vi "外观 2.vi"(0 "Data In":T6 caption="数据输入" format="%04x", 2 "Display State In":T4 caption="显示状态输入", 3 "Container State":T5 caption="容器状态") -> (6 "Data Out":T6 caption="数据输出" format="%04x", 7 "Display State Out":T4 caption="显示状态输出", 8 "Action":T3 caption="动作")   [LabVIEW 2016, in "氨氮调试控件.xctl"]
uses:
  <vilib>/_xctls/Container State.ctl
  <vilib>/_xctls/Action.ctl
  <vilib>/_xctls/XControlSupport.lvlib
panel:
  out "选项卡控件":enum32{"选项卡 1", "选项卡 2"}(tab)
  in  "V9-2":bool
  in  "V9-1":bool
  in  "阀口选择":T1(radio)
  in  "外设":enum32{"未选择", "蠕动泵", "电磁阀1", "电磁阀2", "氨氮控温"}(radio)
  in  "控温":enum32{"未选择", "消解", "恒温", "降温"}(radio)
  in  "灯":enum32{"未选择", "365", "520", "660", "氙灯/紫灯"}(radio)
  in  "ADC值":T2(radio)
  in  "项目输入":enum32{"总磷", "总氮", "氨氮"}(ring)
  in  "功能选择":enum32{"等待", "复位", "注入", "注出"}(radio)=enum."注入"
  in  "数值":i16=4000
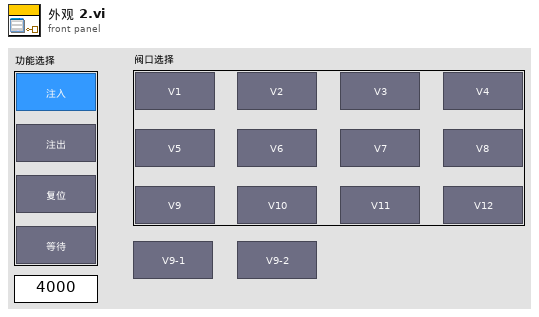
[diagram p1: front panel]
types:
  T1 = enum32{"未选择", "V1", "V2", "V3", "V4", "V5", "V6", "V7", "V8", "V9", "V10", "V11", "V12"}
  T2 = enum32{"未选择", "ADC365", "ADC520", "ADC660", "光谱仪"}
  T3 = typedef "XControlSupport.lvlib/Action.ctl" = cluster{"Data Changed?":bool, "State Changed?":bool, "Action Name":string}
  T4 = typedef "氨氮调试控件.xctl/状态 2.ctl" = cluster{"Numeric":dbl}
  T5 = typedef "XControlSupport.lvlib/Container State.ctl" = cluster{"Indicator?":bool, "Run Mode?":bool, " Refnum":refnum<vi>}
  T6 = typedef "氨氮调试控件.xctl/数据 2.ctl" = u16[]
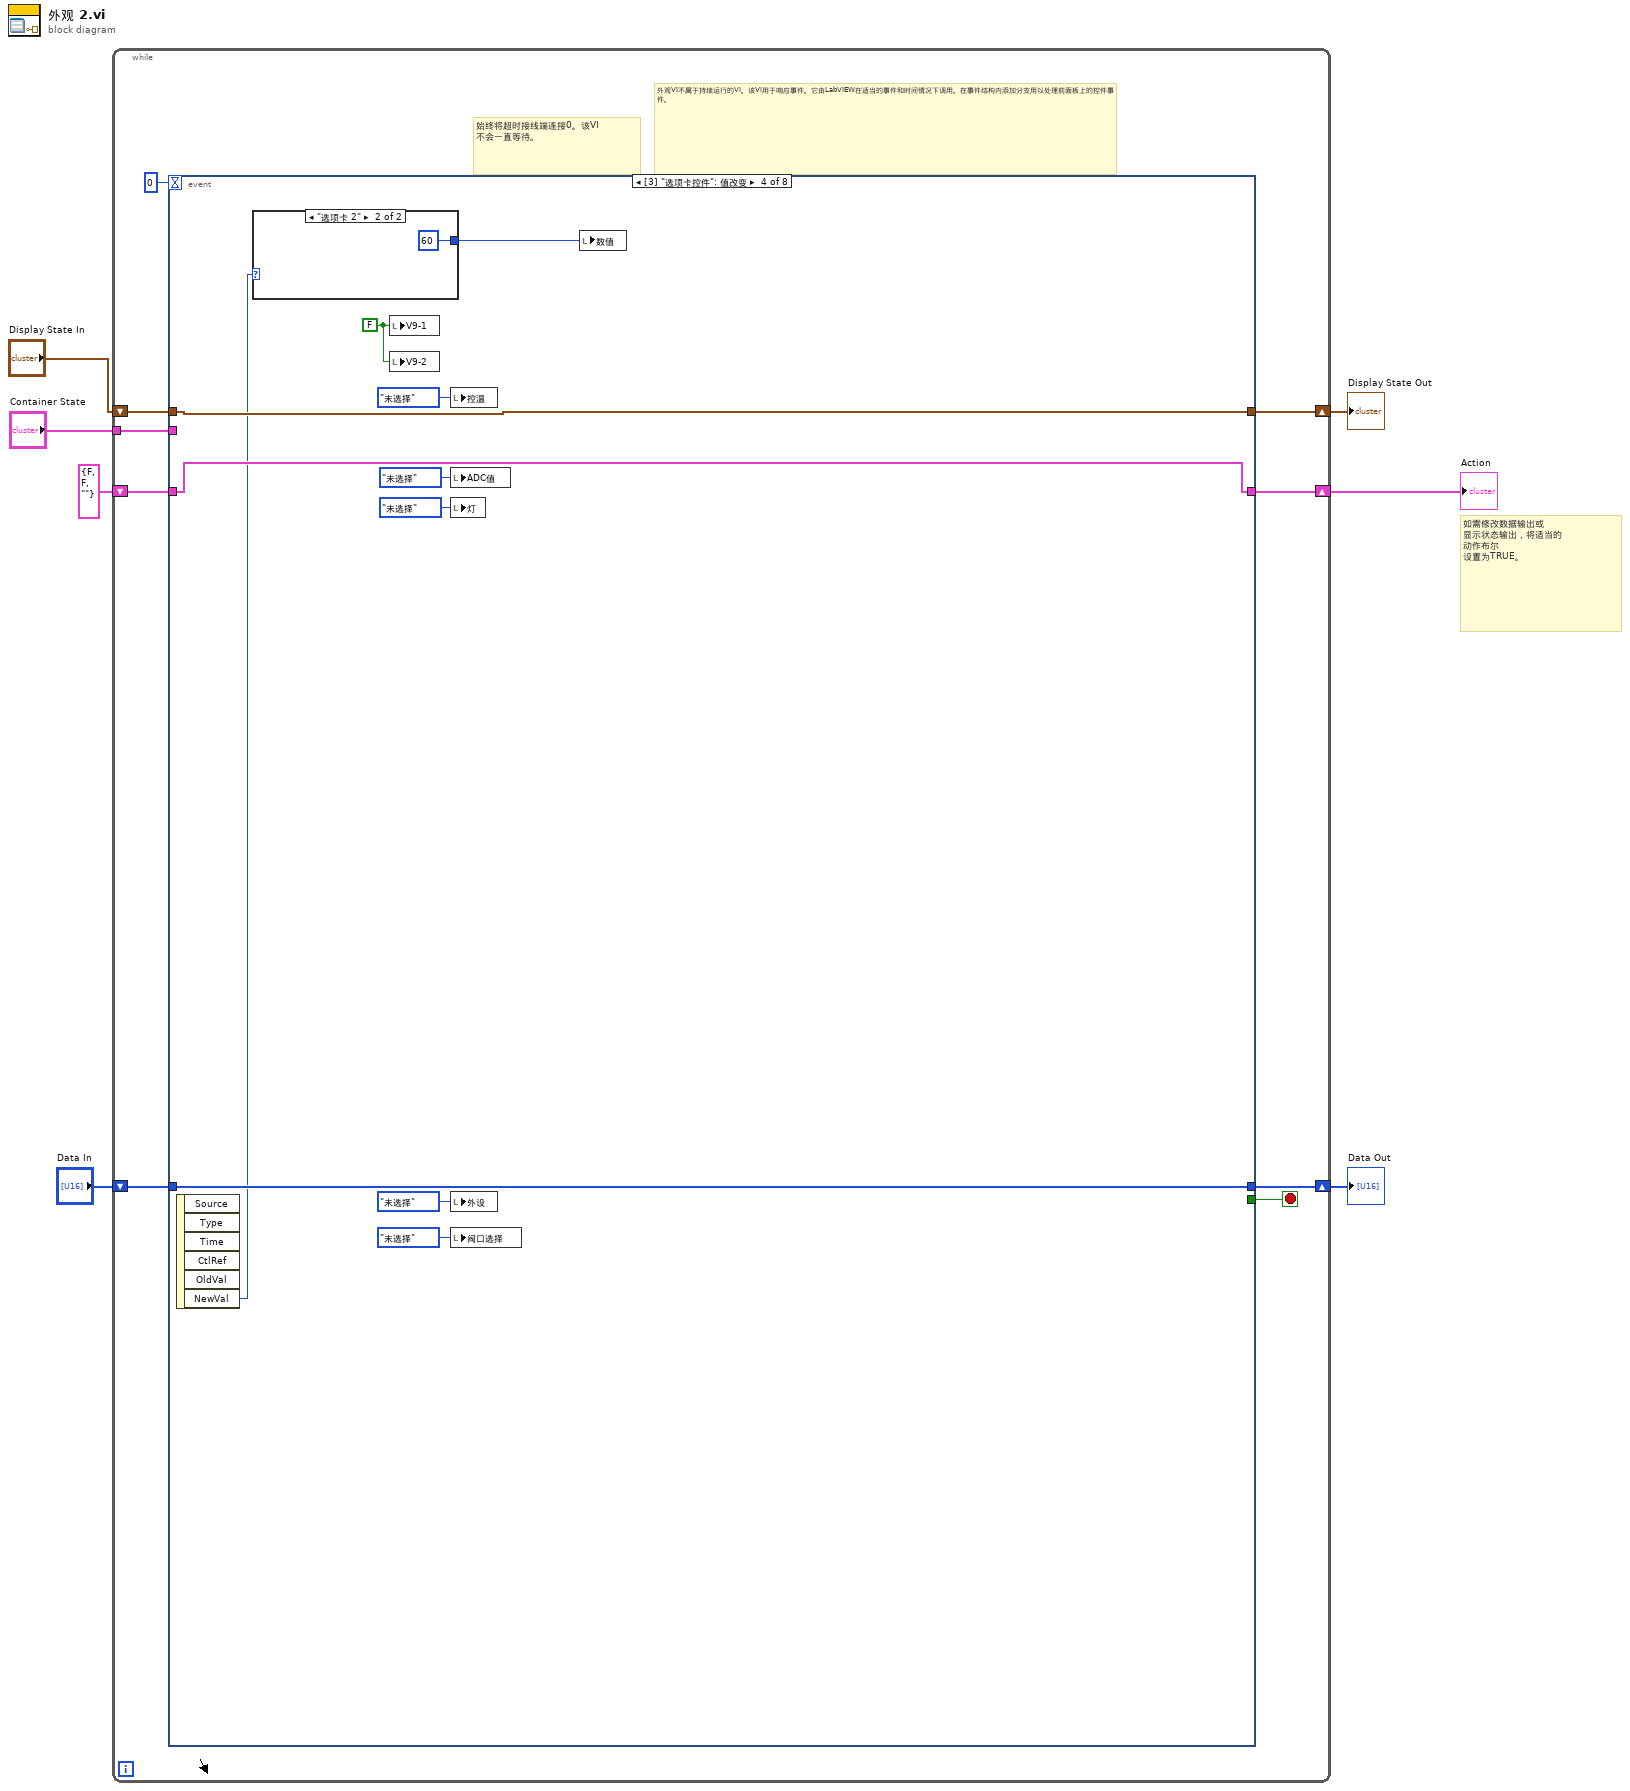
[diagram p0: block diagram]
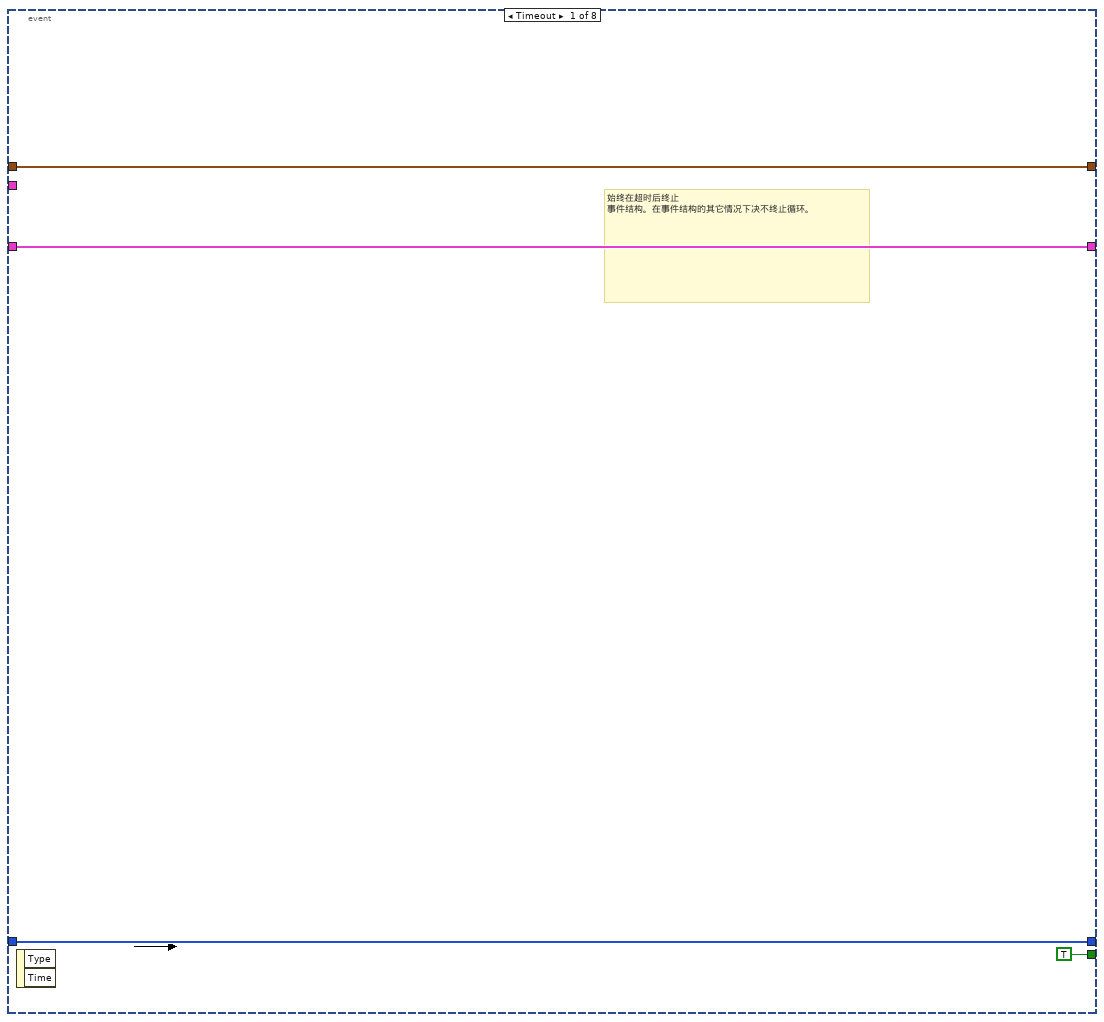
[diagram p2: hidden frame]
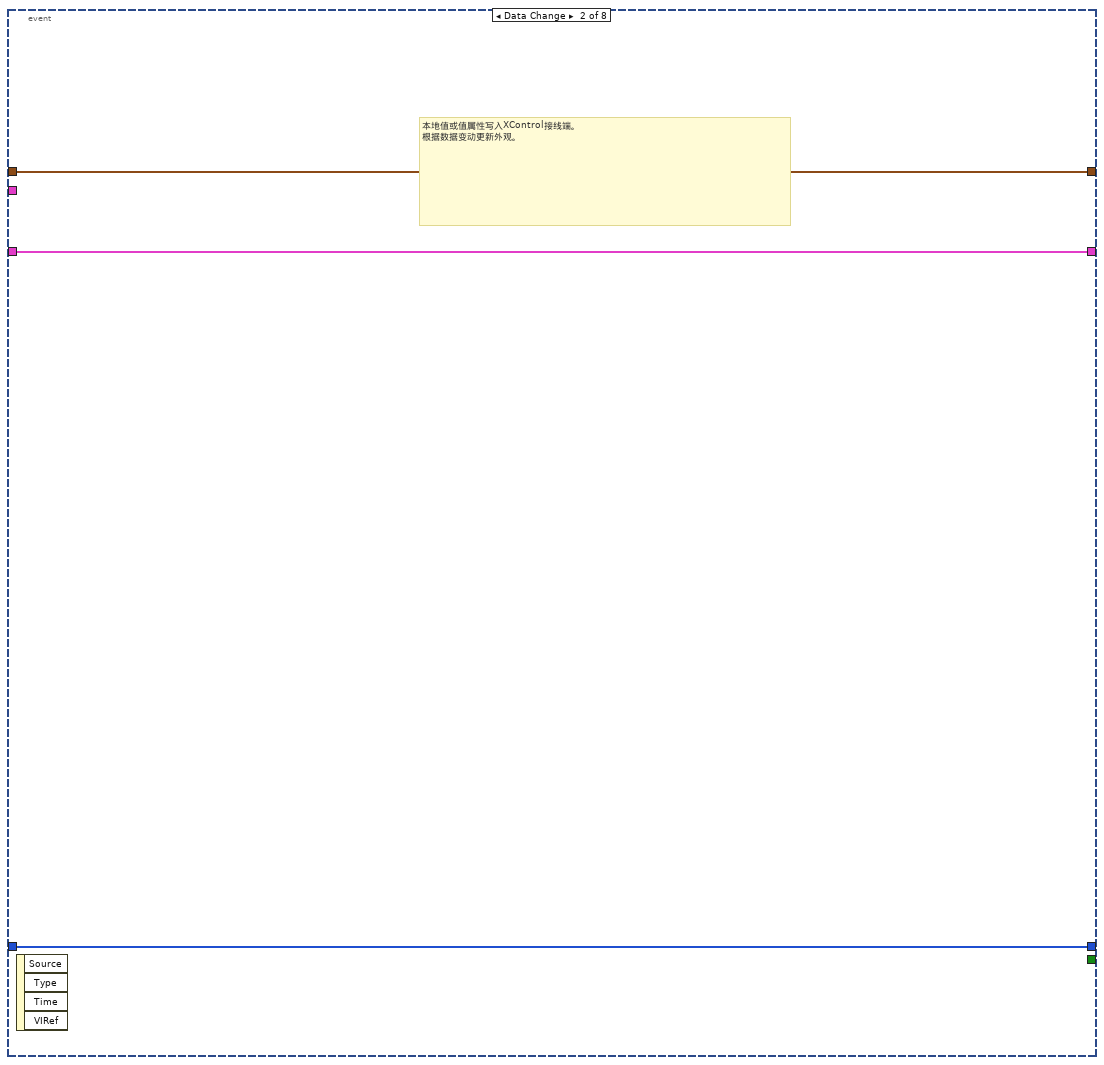
[diagram p3: hidden frame]
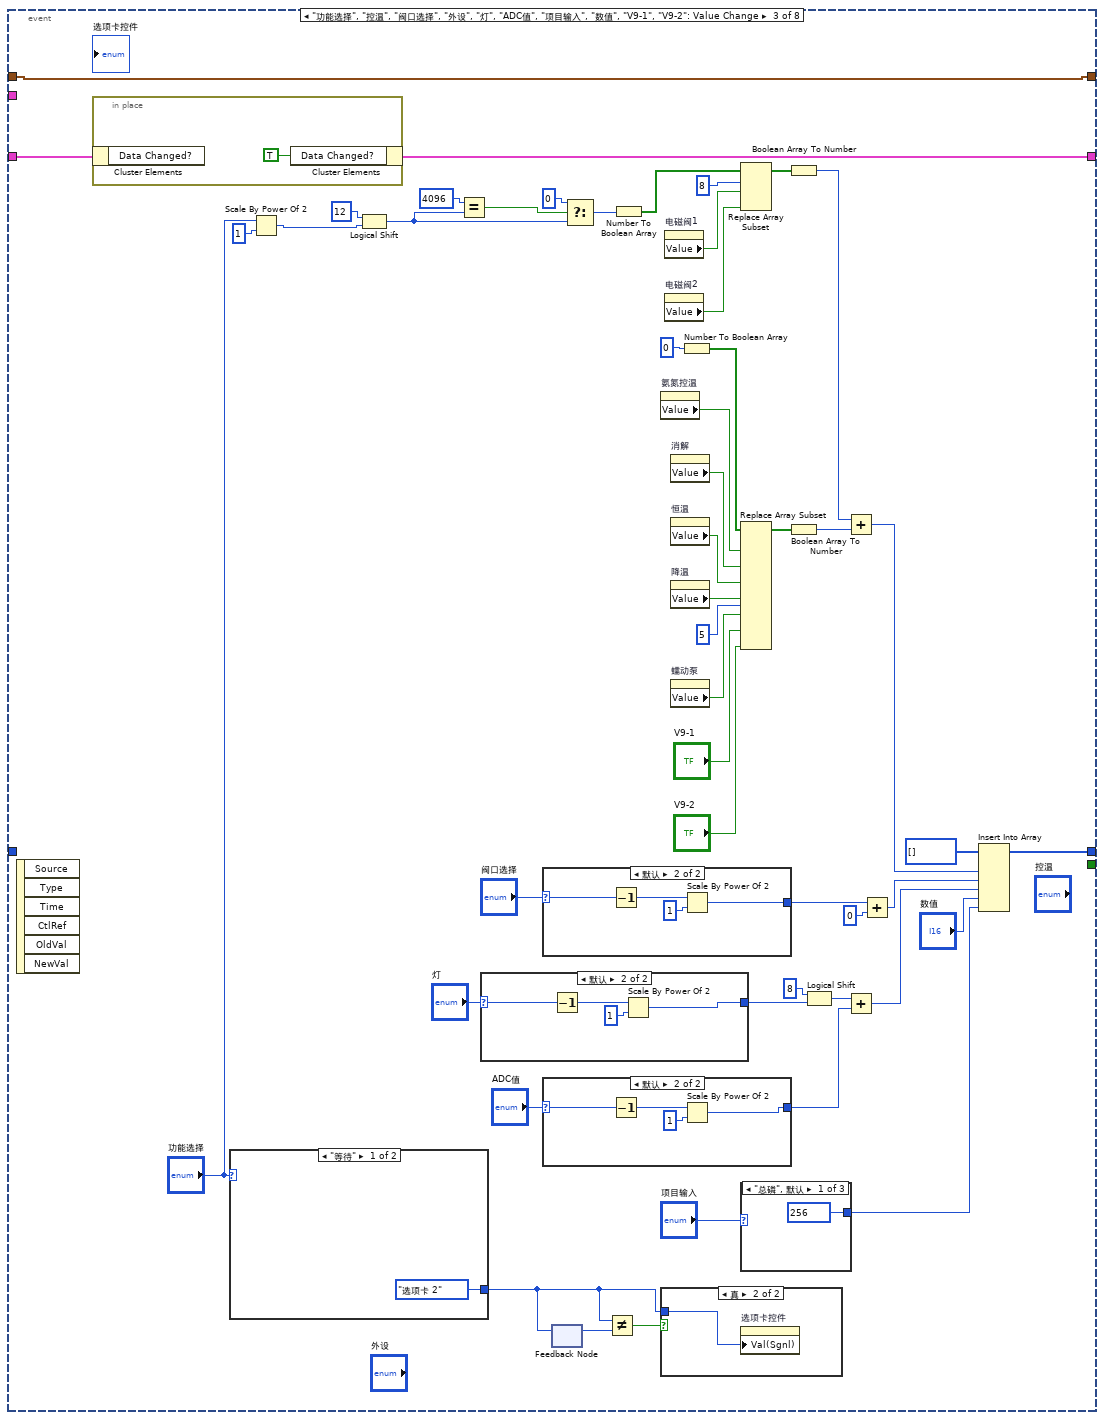
[diagram p4: hidden frame]
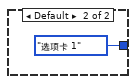
[diagram p6: hidden frame]
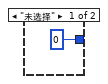
[diagram p7: hidden frame]
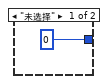
[diagram p8: hidden frame]
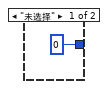
[diagram p9: hidden frame]
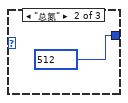
[diagram p10: hidden frame]
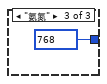
[diagram p11: hidden frame]
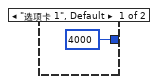
[diagram p12: hidden frame]
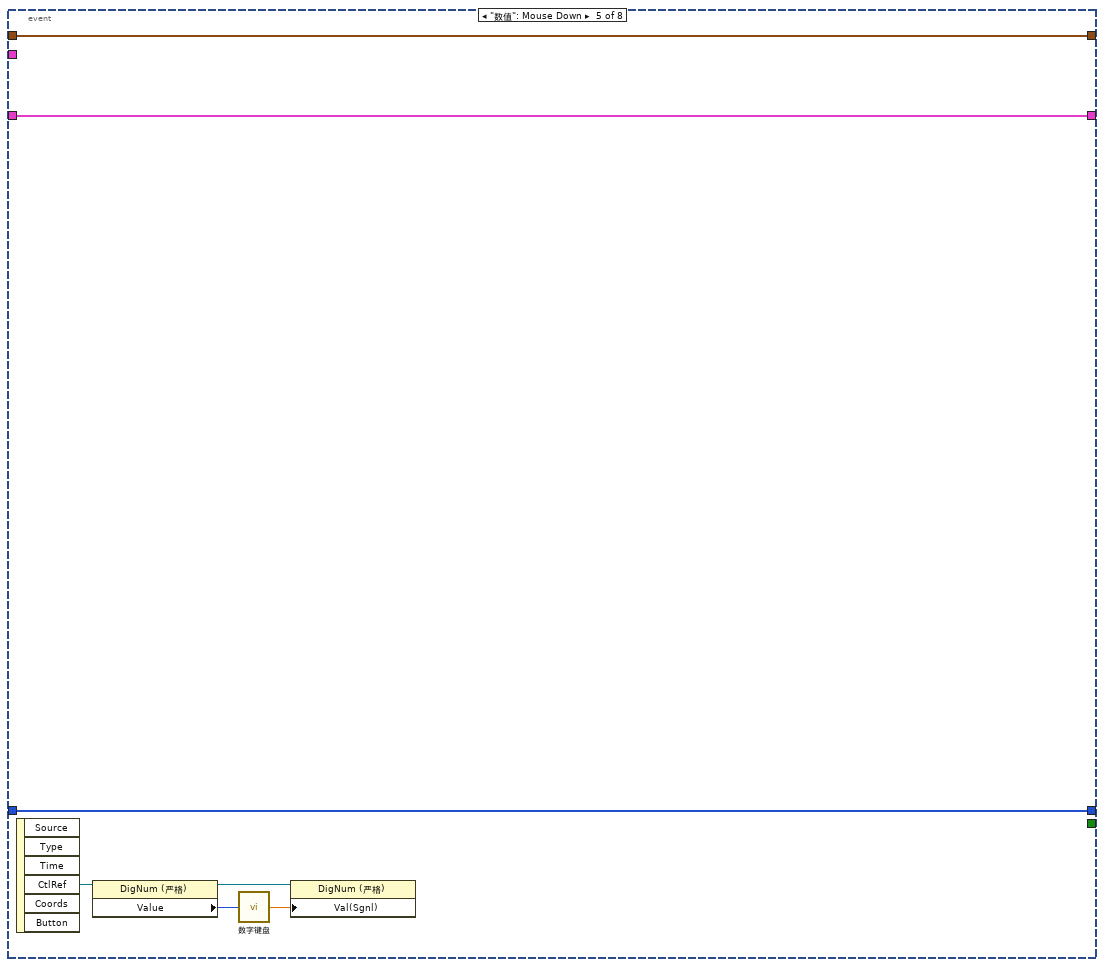
[diagram p13: hidden frame]
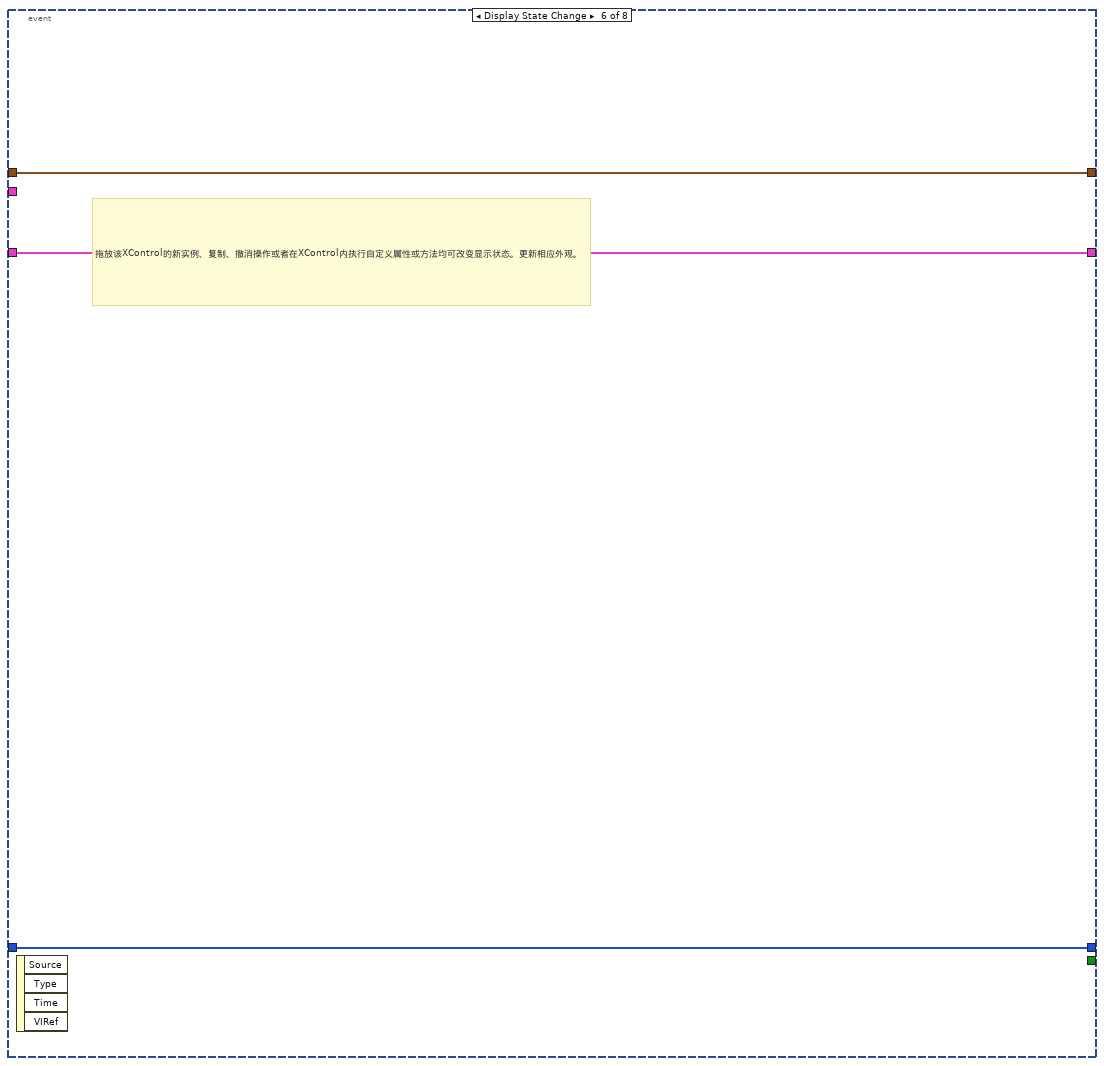
[diagram p14: hidden frame]
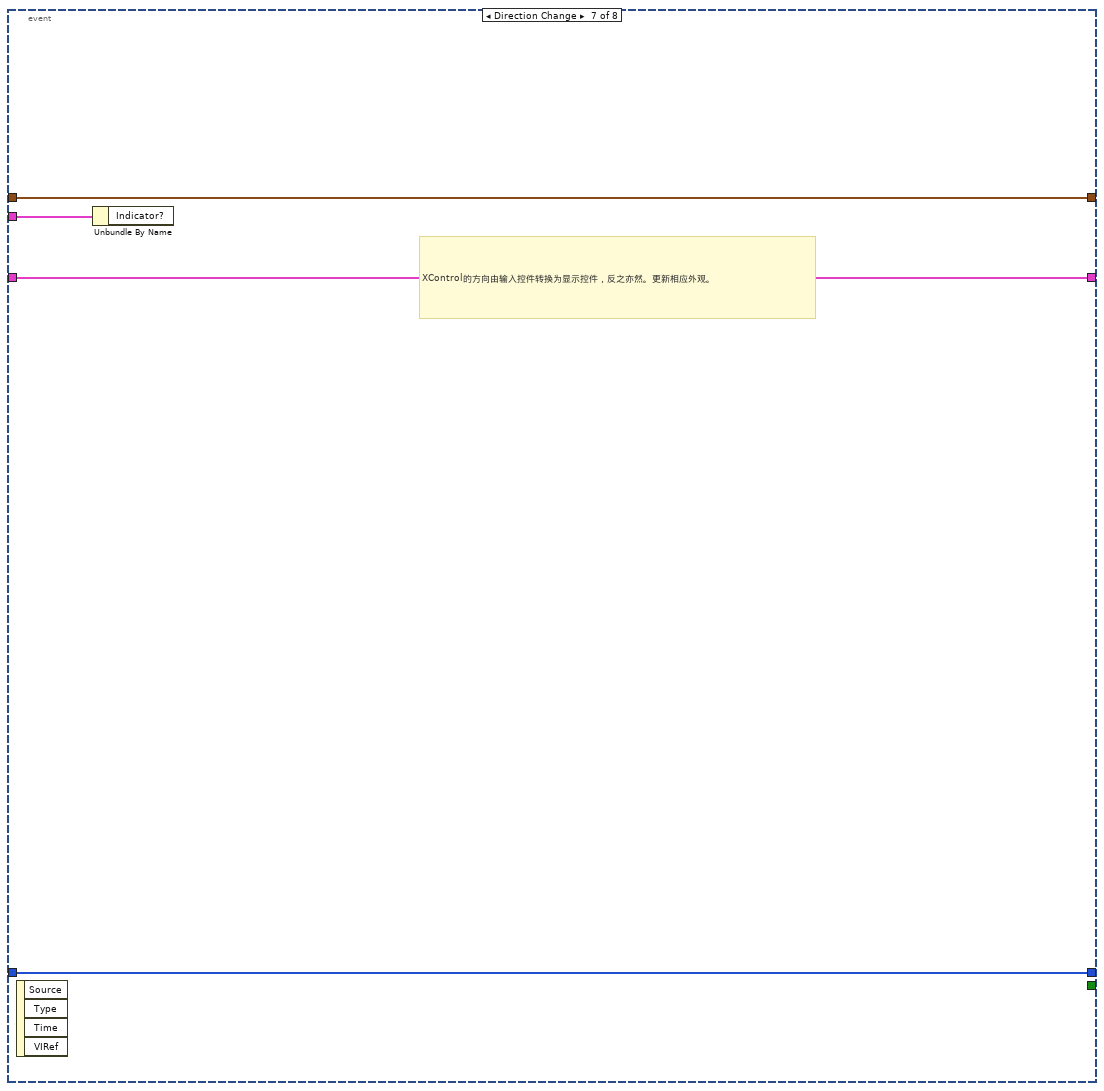
[diagram p15: hidden frame]
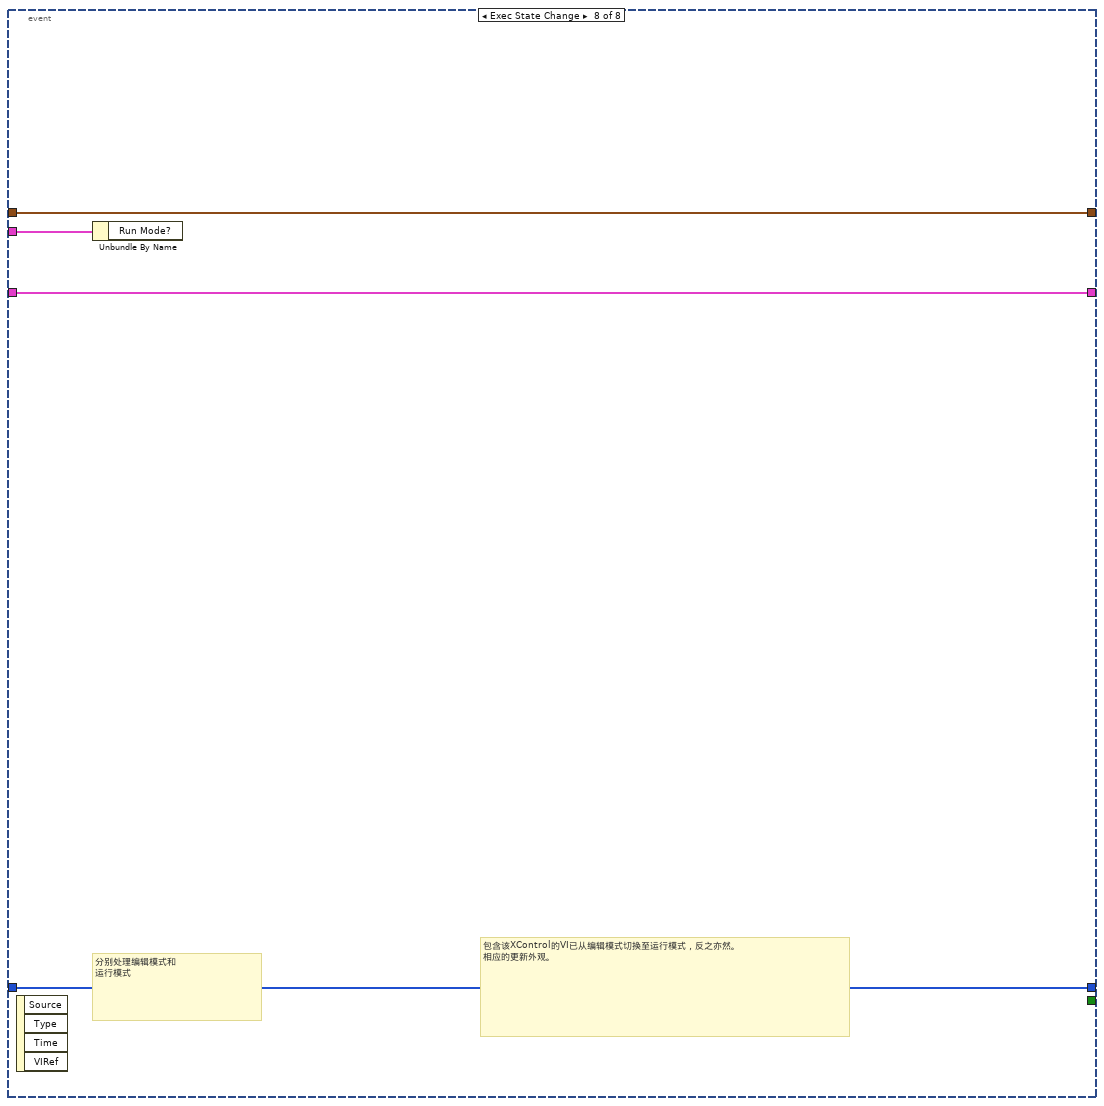
[diagram p16: hidden frame]
diagram:
  # "如需修改数据输出或\n显示状态输出，将适当的\n动作布尔\n设置为TRUE。"
  n1 = while {
    shift-right: [w15] -> w4
    shift-left: "Display State In" -> [w16]
    tunnel: "Container State" -> [w12]
    shift-right: [w10] -> w7
    shift-left: "Data In" -> [w11]
    shift-right: [w8] -> w2
    shift-left: T3 {"Data Changed?"=FALSE, "State Changed?"=FALSE, "Action Name"=""} ("Action") -> [w9]
    stop <- w14 stop-if-true
    # "外观VI不属于持续运行的VI。该VI用于响应事件。它由LabVIEW在适当的事件和时间情况下调用。在事件结构内添加分支用以处理前面板上的控件事件。"
    # "始终将超时接线端连接0。该VI\n不会一直等待。"
    n2 = event shown="[3] \"选项卡控件\": 值改变" {
      selector: _ -> [_ _ _ _ _ _ _ _]
      dyn-events: _ -> [_ _ _ _ _ _ _ _]
      timeout: 0 -> [_ _ _ _ _ _ _ _]
      tunnel: w16 -> [w18 w22 w73 w106 w115 w118 w121 w125]
      tunnel: [w18 w22 w73 w106 w115 w118 w121 w125] -> w15
      tunnel: [TRUE _ _ _ _ _ _ _] -> w14
      tunnel: w12 -> [_ _ _ _ _ _ w122 w126]
      tunnel: w11 -> [w17 w23 _ w105 w114 w117 w120 w124]
      tunnel: [w17 w23 w48 w105 w114 w117 w120 w124] -> w10
      tunnel: [w19 w21 w71 w104 w113 w116 w119 w123] -> w8
      tunnel: w9 -> [w19 w21 w72 w104 w113 w116 w119 w123]
      event Timeout {
        # "始终在超时后终止\n事件结构。在事件结构的其它情况下决不终止循环。"
        n3 = event-data() -> ()  [unwired: 1 in, 2 out]
      }
      event Data Change {
        # "本地值或值属性写入XControl接线端。\n根据数据变动更新外观。"
        n4 = event-data() -> ()  [unwired: 1 in, 4 out]
      }
      event "功能选择", "控温", "阀口选择", "外设", "灯", "ADC值", "项目输入", "数值", "V9-1", "V9-2": Value Change {
        n5 = event-data() -> ()  [unwired: 1 in, 6 out]
        n6 = in-place {
          n7 = in-place-cluster #1(w72) -> ()  [unwired: 1 out]
          n8 = in-place-cluster #1("Data Changed?"=TRUE) -> (w71:T3)
        }
        n9 = case shown="\"等待\"" "功能选择" {
          tunnel: [enum32{"选项卡 1", "选项卡 2"}."选项卡 2" ("选项卡控件") enum32{"选项卡 1", "选项卡 2"}."选项卡 1" ("选项卡控件")] -> w42
          frame "等待" {
          }
          frame Default {
          }
        }
        n10 = Scale By Power Of 2(n="功能选择", x=i16 1 ("y")) -> (x*2^n=w57:i16)
        n11 = Logical Shift(y=i16 12, x=w57) -> (x << y=w62:i16)
        n12 = Equal?(x=u32 4096 ("t"), y=w62) -> (x = y?=w70:bool)
        n13 = case shown="默认" "灯" {
          selector: "灯" -> [_ w84]
          tunnel: [i16 0 ("y") w86] -> w53
          frame "未选择" {
          }
          frame Default {
            n14 = Decrement(x=w84) -> (x-1=w85:enum32{"未选择", "365", "520", "660", "氙灯/紫灯"})
            n15 = Scale By Power Of 2(n=w85, x=i16 1 ("y")) -> (x*2^n=w86:i16)
          }
        }
        n16 = case shown="默认" "阀口选择" {
          selector: "阀口选择" -> [_ w89]
          tunnel: [i16 0 ("y") w91] -> w56
          frame "未选择" {
          }
          frame Default {
            n17 = Decrement(x=w89) -> (x-1=w90:T1)
            n18 = Scale By Power Of 2(n=w90, x=i16 1 ("y")) -> (x*2^n=w91:i16)
          }
        }
        n19 = case shown="默认" "ADC值" {
          selector: "ADC值" -> [_ w79]
          tunnel: [i16 0 ("y") w81] -> w52
          frame "未选择" {
          }
          frame Default {
            n20 = Decrement(x=w79) -> (x-1=w80:T2)
            n21 = Scale By Power Of 2(n=w80, x=i16 1 ("y")) -> (x*2^n=w81:i16)
          }
        }
        n22 = feedback-in #2(w42) -> ()
        n23 = feedback #2() -> (w44:enum32{"选项卡 1", "选项卡 2"})  [unwired: 1 in]
        n24 = Select(t=u32 0, s=w70, f=w62) -> (s? t:f=w37:u32)
        n25 = Not Equal?(x=w42, y=w44) -> (x != y?=w43:bool)
        n26 = Number To Boolean Array(number=w37) -> (Boolean array=w36:bool[])
        n27 = property on="氨氮控温" class="Bool (严格)"() -> ("Value"=w31:bool)  [unwired: 2 in, 2 out]
        n28 = case shown="真" w43 {
          tunnel: w42 -> [_ w74]
          frame False {
          }
          frame True {
            n29 = property on="选项卡控件" class="TabCtl (严格)"("Val(Sgnl)"=w74) -> ()  [unwired: 2 in, 2 out]
          }
        }
        n30 = property on="电磁阀1" class="Bool (严格)"() -> ("Value"=w32:bool)  [unwired: 2 in, 2 out]
        n31 = property on="电磁阀2" class="Bool (严格)"() -> ("Value"=w27:bool)  [unwired: 2 in, 2 out]
        n32 = property on="消解" class="Bool (严格)"() -> ("Value"=w30:bool)  [unwired: 2 in, 2 out]
        n33 = property on="恒温" class="Bool (严格)"() -> ("Value"=w29:bool)  [unwired: 2 in, 2 out]
        n34 = property on="降温" class="Bool (严格)"() -> ("Value"=w28:bool)  [unwired: 2 in, 2 out]
        n35 = property on="蠕动泵" class="Bool (严格)"() -> ("Value"=w38:bool)  [unwired: 2 in, 2 out]
        n36 = Number To Boolean Array(number=u16 0) -> (Boolean array=w24:bool[])
        n37 = Replace Array Subset(array=w36, new element #1=w32, index #1=8 ("索引"), new element #2=w27) -> (w35:bool[])  [unwired: 1 in]
        n38 = Replace Array Subset(array=w24, new element #1=w31, new element #2=w30, new element #3=w29, new element #4=w28, new element #5=w38, index #5=5 ("索引"), new element #6="V9-1", new element #7="V9-2") -> (w45:bool[])  [unwired: 6 in]
        n39 = case shown="\"总磷\", 默认" "项目输入" {
          tunnel: [256 512 768] -> w59
          frame "总磷", Default {
          }
          frame "总氮" {
          }
          frame "氨氮" {
          }
        }
        n40 = Boolean Array To Number(Boolean array=w35) -> (number=w34:u32)
        n41 = Boolean Array To Number(Boolean array=w45) -> (number=w41:u32)
        n42 = Logical Shift(y=i16 8, x=w53) -> (x << y=w68:i16)
        n43 = Add(x=w34, y=w41) -> (x+y=w65:u32)
        n44 = Add(x=w68, y=w52) -> (x+y=w64:i16)
        n45 = Add(x=w56, y=i16 0) -> (x+y=w55:i16)
        n46 = Insert Into Array(array=u16[] [] ("数组"), new element #1=w65, new element #2=w55, new element #3=w64, new element #4="数值", new element #5=w59) -> (w48:u16[])  [unwired: 1 in]
      }
      event "选项卡控件": Value Change {
        w98 = FALSE ("V9-1")
        n47 = event-data() -> ("NewVal"=w103:enum32{"选项卡 1", "选项卡 2"})  [unwired: 1 in, 5 out]
        n48 = case shown="\"选项卡 2\"" w103 {
          tunnel: [i16 4000 ("数值") i16 60 ("数值")] -> w102
          frame "选项卡 1", Default {
          }
          frame "选项卡 2" {
          }
        }
        n49 = local write "V9-1"(w98) -> ()
        n50 = local write "V9-2"(w98) -> ()
        n51 = local write "控温"(enum32{"未选择", "消解", "恒温", "降温"}."未选择" ("控温")) -> ()
        n52 = local write "ADC值"(T2."未选择" ("ADC值")) -> ()
        n53 = local write "灯"(enum32{"未选择", "365", "520", "660", "氙灯/紫灯"}."未选择" ("灯")) -> ()
        n54 = local write "外设"(enum32{"未选择", "蠕动泵", "电磁阀1", "电磁阀2", "氨氮控温"}."未选择" ("外设")) -> ()
        n55 = local write "阀口选择"(T1."未选择" ("阀口选择")) -> ()
        n56 = local write "数值"(w102) -> ()
      }
      event "数值": Mouse Down {
        n57 = event-data() -> ("CtlRef"=w112:refnum<vi>)  [unwired: 1 in, 5 out]
        n58 = property class="DigNum (严格)"(reference=w112) -> (reference out=w111:refnum<vi>, "Value"=w110:i16)  [unwired: 1 in, 1 out]
        n59 = call "数字键盘.vi"("OldNumber"=w110) -> ("NewNumber"=w109:sgl)
        n60 = property class="DigNum (严格)"(reference=w111, "Val(Sgnl)"=w109) -> ()  [unwired: 1 in, 2 out]
      }
      event Display State Change {
        # "拖放该XControl的新实例、复制、撤消操作或者在XControl内执行自定义属性或方法均可改变显示状态。更新相应外观。"
        n61 = event-data() -> ()  [unwired: 1 in, 4 out]
      }
      event Direction Change {
        # "XControl的方向由输入控件转换为显示控件，反之亦然。更新相应外观。"
        n62 = event-data() -> ()  [unwired: 1 in, 4 out]
        n63 = Unbundle By Name(w122) -> ()  [unwired: 1 out]
      }
      event Exec State Change {
        # "包含该XControl的VI已从编辑模式切换至运行模式，反之亦然。\n相应的更新外观。"
        # "分别处理编辑模式和\n运行模式"
        n64 = event-data() -> ()  [unwired: 1 in, 4 out]
        n65 = Unbundle By Name(w126) -> ()  [unwired: 1 out]
      }
    }
  }
  "Display State Out" <- w4
  "Data Out" <- w7
  "Action" <- w2
